vi "LS370Monitor.vi"() -> ()   [LabVIEW 2019]
uses:
  Utility/LS370/Monitor/LS370_Status.ctl
  Instrument_Setup.vi
  Global/Global Variables/global.vi
  Global/Global Variables/Data_Display_global.vi
  Utility/Monitor Communication/sub-vis/LS370_Open_Queue.vi
panel:
  out "Lakeshore 370":T1
  out "Tsweeps Running":bool
  in  "Stopp":bool
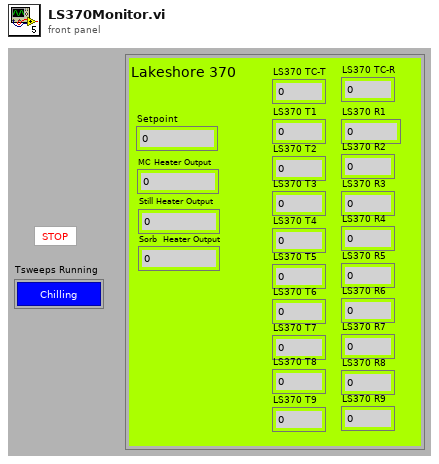
[diagram p1: front panel]
types:
  T1 = typedef "LS370_Status.ctl" = cluster{"Setpoint":dbl, "MC Heater Output":dbl, "Still Heater Output":dbl, "Sorb  Heater Output":dbl, "LS370 T1":dbl, "LS370 T2":dbl, "LS370 T3":dbl, "LS370 T4":dbl, "LS370 T5":dbl, "LS370 R1":dbl, "LS370 R2":dbl, "LS370 R3":dbl, "LS370 R4":dbl, "LS370 R5":dbl, "LS370 T6":dbl, "LS370 T7":dbl, "LS370 T8":dbl, "LS370 T9":dbl, "LS370 R6":dbl, "LS370 R7":dbl, "LS370 R8":dbl, "LS370 R9":dbl, "LS370 TC-T":dbl, "LS370 TC-R":dbl}
  T2 = typedef "LS370-Control.ctl" = cluster{"Disable Heater":bool, "Activate Tsweep":bool, "Update Lakeshores":bool, "Setpoint - Manual":dbl, "Rate (K/min)":dbl, "Sorb Power (mW)":dbl, "Still Power (mW)":dbl, "Sorb Heater":bool, "Still Heater":bool, "Set Temperature Sweep Main":bool}
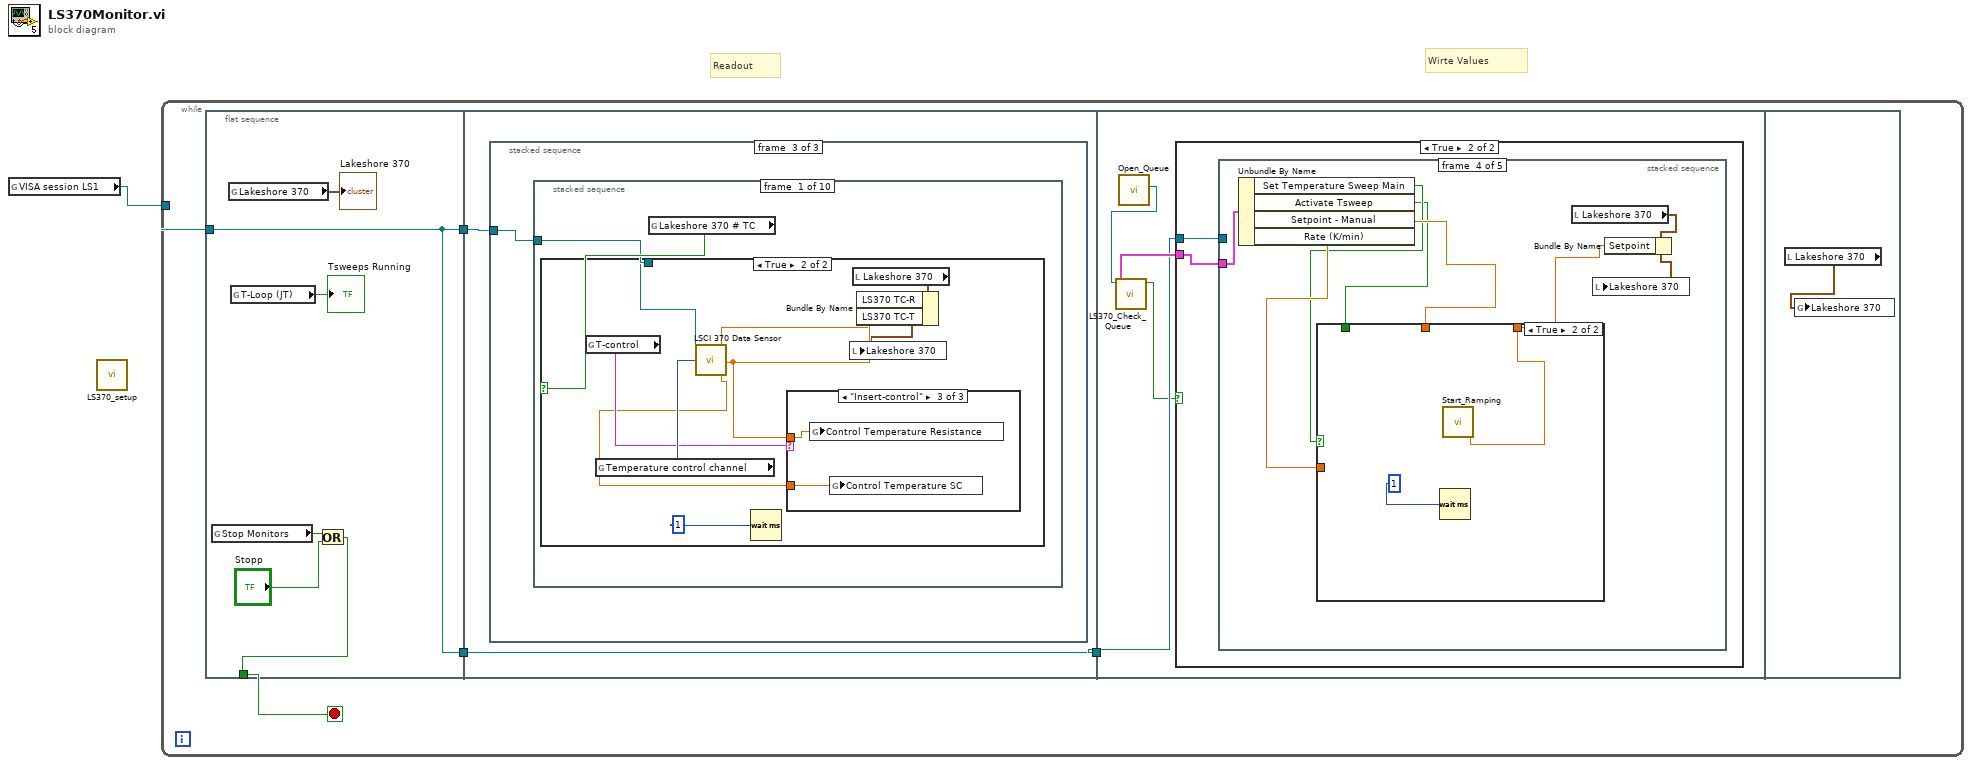
[diagram p0: block diagram]
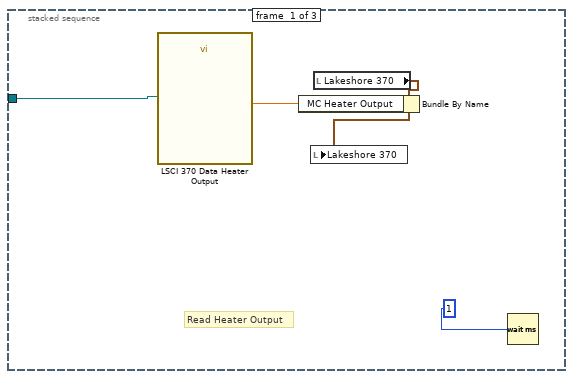
[diagram p2: hidden frame]
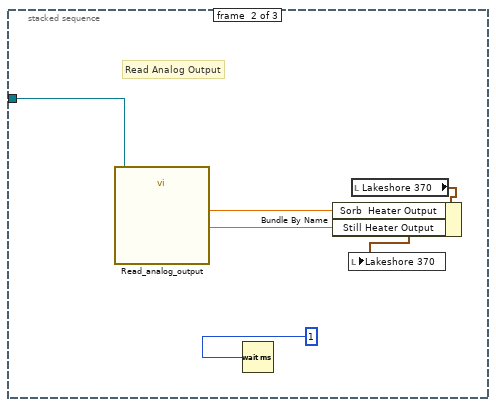
[diagram p3: hidden frame]
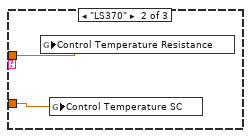
[diagram p6: hidden frame]
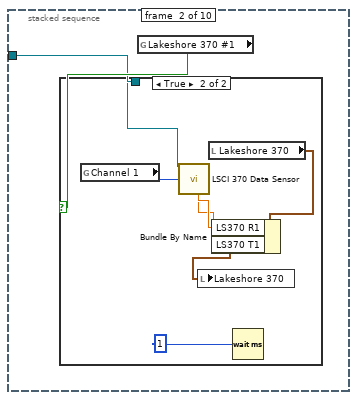
[diagram p7: hidden frame]
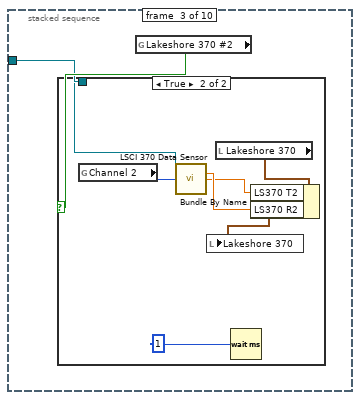
[diagram p9: hidden frame]
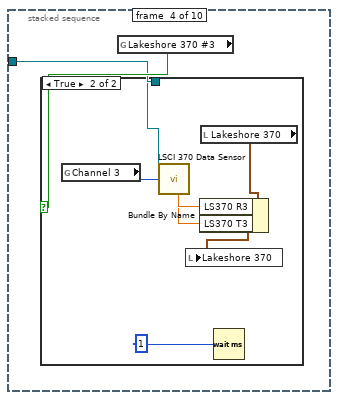
[diagram p11: hidden frame]
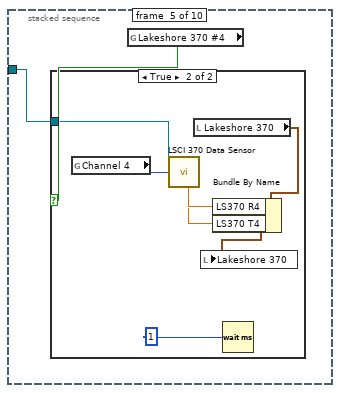
[diagram p13: hidden frame]
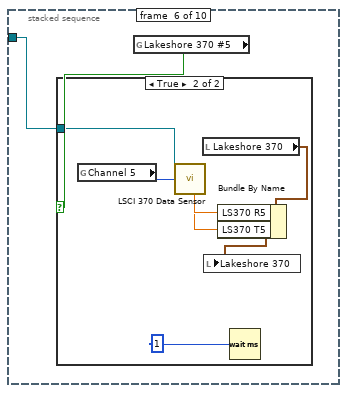
[diagram p15: hidden frame]
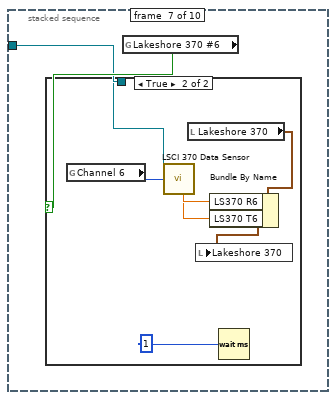
[diagram p17: hidden frame]
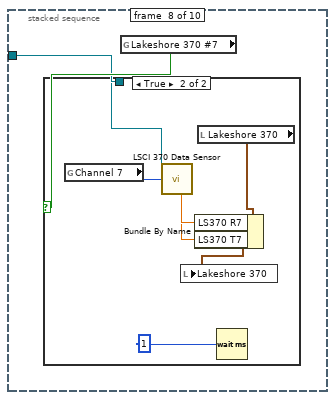
[diagram p19: hidden frame]
diagram:
  # "Wirte Values"
  # "Readout"
  n1 = global read "Instrument_Setup.vi" "VISA session LS1"() -> (w1:refnum<visa-resource-name>)
  n2 = call "LS370_setup.vi"() -> ()  [unwired: 1 in]
  n3 = while {
    tunnel: w1 -> [w5]
    stop <- w2 stop-if-true
    n4 = flat-sequence {
      tunnel: w5 -> [w8]
      tunnel: [w8] -> w6
      tunnel: [w8] -> w3
      tunnel: [w7] -> w2
      tunnel: w6 -> [w14]
      tunnel: [w13] -> w4
      tunnel: w3 -> [w13]
      tunnel: w4 -> [w124]
      frame #0 {
        n5 = global read "Data_Display_global.vi" "Stop Monitors"() -> (w10:bool)
        n6 = global read "Data_Display_global.vi" "Lakeshore 370"() -> (→"Lakeshore 370":T1)
        n7 = global read "global.vi" "T-Loop (JT)"() -> (→"Tsweeps Running":bool)
        n8 = Or(x=w10, y="Stopp") -> (x .or. y?=w7:bool)
      }
      frame #1 {
        n9 = stacked-sequence {
          tunnel: w14 -> [w19 w25 w26]
          frame #0 {
            # "Read Heater Output"
            n10 = call "LSCI 370 Data Heater Output.vi"("VISA session"=w19) -> ("Heater Output"=w16:dbl)  [unwired: 12 in, 2 out]
            n11 = local read "Lakeshore 370"() -> (w17:T1)
            n12 = Bundle By Name(cluster=w17, "MC Heater Output"=w16) -> (w15:T1)
            n13 = local write "Lakeshore 370"(w15) -> ()
            n14 = Wait (ms)(milliseconds to wait=1) -> ()  [unwired: 1 out]
          }
          frame #1 {
            # "Read Analog Output"
            n15 = call "Read_analog_output.vi"("VISA session"=w25) -> ("Still Output"=w20:dbl, "Analog Output"=w21:dbl)  [unwired: 9 in]
            n16 = Wait (ms)(milliseconds to wait=1) -> ()  [unwired: 1 out]
            n17 = local read "Lakeshore 370"() -> (w23:T1)
            n18 = Bundle By Name(cluster=w23, "Sorb  Heater Output"=w21, "Still Heater Output"=w20) -> (w22:T1)
            n19 = local write "Lakeshore 370"(w22) -> ()
          }
          frame #2 {
            n20 = stacked-sequence {
              tunnel: w26 -> [w27 w41 w50 w59 w68 w77 w86 w95 w104 w113]
              frame #0 {
                n21 = global read "Instrument_Setup.vi" "Lakeshore 370 # TC"() -> (w28:bool)
                n22 = case shown="True" w28 {
                  tunnel: w27 -> [_ w34]
                  frame False {
                  }
                  frame True {
                    n23 = global read "Instrument_Setup.vi" "T-control"() -> (w33:string)
                    n24 = global read "Instrument_Setup.vi" "Temperature control channel"() -> (w36:i32)
                    n25 = call "LSCI 370 Data Sensor.vi"("VISA session"=w34, "Channel (1)"=w36) -> ("Resistance Reading"=w31:dbl, "Kelvin Reading"=w30:dbl)  [unwired: 9 in, 3 out]
                    n26 = Wait (ms)(milliseconds to wait=1) -> ()  [unwired: 1 out]
                    n27 = case shown="\"Insert-control\"" w33 {
                      tunnel: w31 -> [_ w38 w40]
                      tunnel: w30 -> [_ w37 w39]
                      frame "None", Default {
                      }
                      frame "LS370" {
                        n28 = global write "Data_Display_global.vi" "Control Temperature Resistance"(w38) -> ()
                        n29 = global write "Data_Display_global.vi" "Control Temperature SC"(w37) -> ()
                      }
                      frame "Insert-control" {
                        n30 = global write "Data_Display_global.vi" "Control Temperature Resistance"(w40) -> ()
                        n31 = global write "Data_Display_global.vi" "Control Temperature SC"(w39) -> ()
                      }
                    }
                    n32 = local read "Lakeshore 370"() -> (w32:T1)
                    n33 = Bundle By Name(cluster=w32, "LS370 TC-R"=w31, "LS370 TC-T"=w30) -> (w29:T1)
                    n34 = local write "Lakeshore 370"(w29) -> ()
                  }
                }
              }
              frame #1 {
                n35 = global read "Instrument_Setup.vi" "Lakeshore 370 #1"() -> (w42:bool)
                n36 = case shown="True" w42 {
                  tunnel: w41 -> [_ w47]
                  frame False {
                  }
                  frame True {
                    n37 = global read "Instrument_Setup.vi" "Channel 1"() -> (w49:i32)
                    n38 = call "LSCI 370 Data Sensor.vi"("VISA session"=w47, "Channel (1)"=w49) -> ("Resistance Reading"=w44:dbl, "Kelvin Reading"=w43:dbl)  [unwired: 9 in, 3 out]
                    n39 = local read "Lakeshore 370"() -> (w46:T1)
                    n40 = Bundle By Name(cluster=w46, "LS370 R1"=w44, "LS370 T1"=w43) -> (w45:T1)
                    n41 = local write "Lakeshore 370"(w45) -> ()
                    n42 = Wait (ms)(milliseconds to wait=1) -> ()  [unwired: 1 out]
                  }
                }
              }
              frame #2 {
                n43 = global read "Instrument_Setup.vi" "Lakeshore 370 #2"() -> (w51:bool)
                n44 = case shown="True" w51 {
                  tunnel: w50 -> [_ w56]
                  frame False {
                  }
                  frame True {
                    n45 = global read "Instrument_Setup.vi" "Channel 2"() -> (w58:i32)
                    n46 = call "LSCI 370 Data Sensor.vi"("VISA session"=w56, "Channel (1)"=w58) -> ("Resistance Reading"=w53:dbl, "Kelvin Reading"=w52:dbl)  [unwired: 9 in, 3 out]
                    n47 = local read "Lakeshore 370"() -> (w55:T1)
                    n48 = Wait (ms)(milliseconds to wait=1) -> ()  [unwired: 1 out]
                    n49 = Bundle By Name(cluster=w55, "LS370 T2"=w52, "LS370 R2"=w53) -> (w54:T1)
                    n50 = local write "Lakeshore 370"(w54) -> ()
                  }
                }
              }
              frame #3 {
                n51 = global read "Instrument_Setup.vi" "Lakeshore 370 #3"() -> (w60:bool)
                n52 = case shown="True" w60 {
                  tunnel: w59 -> [_ w65]
                  frame False {
                  }
                  frame True {
                    n53 = global read "Instrument_Setup.vi" "Channel 3"() -> (w67:i32)
                    n54 = call "LSCI 370 Data Sensor.vi"("VISA session"=w65, "Channel (1)"=w67) -> ("Resistance Reading"=w62:dbl, "Kelvin Reading"=w61:dbl)  [unwired: 9 in, 3 out]
                    n55 = local read "Lakeshore 370"() -> (w64:T1)
                    n56 = Bundle By Name(cluster=w64, "LS370 R3"=w62, "LS370 T3"=w61) -> (w63:T1)
                    n57 = local write "Lakeshore 370"(w63) -> ()
                    n58 = Wait (ms)(milliseconds to wait=1) -> ()  [unwired: 1 out]
                  }
                }
              }
              frame #4 {
                n59 = global read "Instrument_Setup.vi" "Lakeshore 370 #4"() -> (w69:bool)
                n60 = case shown="True" w69 {
                  tunnel: w68 -> [_ w74]
                  frame False {
                  }
                  frame True {
                    n61 = global read "Instrument_Setup.vi" "Channel 4"() -> (w76:i32)
                    n62 = call "LSCI 370 Data Sensor.vi"("VISA session"=w74, "Channel (1)"=w76) -> ("Resistance Reading"=w71:dbl, "Kelvin Reading"=w70:dbl)  [unwired: 9 in, 3 out]
                    n63 = local read "Lakeshore 370"() -> (w73:T1)
                    n64 = Bundle By Name(cluster=w73, "LS370 R4"=w71, "LS370 T4"=w70) -> (w72:T1)
                    n65 = local write "Lakeshore 370"(w72) -> ()
                    n66 = Wait (ms)(milliseconds to wait=1) -> ()  [unwired: 1 out]
                  }
                }
              }
              frame #5 {
                n67 = global read "Instrument_Setup.vi" "Lakeshore 370 #5"() -> (w78:bool)
                n68 = case shown="True" w78 {
                  tunnel: w77 -> [_ w83]
                  frame False {
                  }
                  frame True {
                    n69 = global read "Instrument_Setup.vi" "Channel 5"() -> (w85:i32)
                    n70 = call "LSCI 370 Data Sensor.vi"("VISA session"=w83, "Channel (1)"=w85) -> ("Resistance Reading"=w81:dbl, "Kelvin Reading"=w80:dbl)  [unwired: 9 in, 3 out]
                    n71 = local read "Lakeshore 370"() -> (w82:T1)
                    n72 = Bundle By Name(cluster=w82, "LS370 R5"=w81, "LS370 T5"=w80) -> (w79:T1)
                    n73 = local write "Lakeshore 370"(w79) -> ()
                    n74 = Wait (ms)(milliseconds to wait=1) -> ()  [unwired: 1 out]
                  }
                }
              }
              frame #6 {
                n75 = global read "Instrument_Setup.vi" "Lakeshore 370 #6"() -> (w87:bool)
                n76 = case shown="True" w87 {
                  tunnel: w86 -> [_ w92]
                  frame False {
                  }
                  frame True {
                    n77 = global read "Instrument_Setup.vi" "Channel 6"() -> (w94:i32)
                    n78 = call "LSCI 370 Data Sensor.vi"("VISA session"=w92, "Channel (1)"=w94) -> ("Resistance Reading"=w90:dbl, "Kelvin Reading"=w89:dbl)  [unwired: 9 in, 3 out]
                    n79 = local read "Lakeshore 370"() -> (w91:T1)
                    n80 = Bundle By Name(cluster=w91, "LS370 R6"=w90, "LS370 T6"=w89) -> (w88:T1)
                    n81 = local write "Lakeshore 370"(w88) -> ()
                    n82 = Wait (ms)(milliseconds to wait=1) -> ()  [unwired: 1 out]
                  }
                }
              }
              frame #7 {
                n83 = global read "Instrument_Setup.vi" "Lakeshore 370 #7"() -> (w96:bool)
                n84 = case shown="True" w96 {
                  tunnel: w95 -> [_ w101]
                  frame False {
                  }
                  frame True {
                    n85 = global read "Instrument_Setup.vi" "Channel 7"() -> (w103:i32)
                    n86 = call "LSCI 370 Data Sensor.vi"("VISA session"=w101, "Channel (1)"=w103) -> ("Resistance Reading"=w99:dbl, "Kelvin Reading"=w98:dbl)  [unwired: 9 in, 3 out]
                    n87 = local read "Lakeshore 370"() -> (w100:T1)
                    n88 = Bundle By Name(cluster=w100, "LS370 R7"=w99, "LS370 T7"=w98) -> (w97:T1)
                    n89 = local write "Lakeshore 370"(w97) -> ()
                    n90 = Wait (ms)(milliseconds to wait=1) -> ()  [unwired: 1 out]
                  }
                }
              }
              frame #8 {
                n91 = global read "Instrument_Setup.vi" "Lakeshore 370 #8"() -> (w105:bool)
                n92 = case shown="True" w105 {
                  tunnel: w104 -> [_ w110]
                  frame False {
                  }
                  frame True {
                    n93 = global read "Instrument_Setup.vi" "Channel 8"() -> (w112:i32)
                    n94 = call "LSCI 370 Data Sensor.vi"("VISA session"=w110, "Channel (1)"=w112) -> ("Resistance Reading"=w108:dbl, "Kelvin Reading"=w107:dbl)  [unwired: 9 in, 3 out]
                    n95 = local read "Lakeshore 370"() -> (w109:T1)
                    n96 = Bundle By Name(cluster=w109, "LS370 R8"=w108, "LS370 T8"=w107) -> (w106:T1)
                    n97 = local write "Lakeshore 370"(w106) -> ()
                    n98 = Wait (ms)(milliseconds to wait=1) -> ()  [unwired: 1 out]
                  }
                }
              }
              frame #9 {
                n99 = global read "Instrument_Setup.vi" "Lakeshore 370 #9"() -> (w114:bool)
                n100 = case shown="True" w114 {
                  tunnel: w113 -> [_ w119]
                  frame False {
                  }
                  frame True {
                    n101 = global read "Instrument_Setup.vi" "Channel 9"() -> (w121:i32)
                    n102 = call "LSCI 370 Data Sensor.vi"("VISA session"=w119, "Channel (1)"=w121) -> ("Resistance Reading"=w117:dbl, "Kelvin Reading"=w116:dbl)  [unwired: 9 in, 3 out]
                    n103 = local read "Lakeshore 370"() -> (w118:T1)
                    n104 = Bundle By Name(cluster=w118, "LS370 R9"=w117, "LS370 T9"=w116) -> (w115:T1)
                    n105 = local write "Lakeshore 370"(w115) -> ()
                    n106 = Wait (ms)(milliseconds to wait=1) -> ()  [unwired: 1 out]
                  }
                }
              }
            }
          }
        }
      }
      frame #2 {
        n107 = call-poly "Open_Queue.vi"() -> ("queue out"=w123:refnum<queue>)  [unwired: 10 in, 1 out]
        n108 = call "LS370_Check_Queue.vi"("queue"=w123) -> ("Control"=w125:T2, "New Entries?"=w122:bool)  [unwired: 7 in, 1 out]
        n109 = case shown="True" w122 {
          tunnel: w125 -> [_ w126]
          tunnel: w124 -> [_ w127]
          frame False {
          }
          frame True {
            n110 = stacked-sequence {
              tunnel: w127 -> [w133 w139 _ _ _]
              tunnel: w126 -> [w130 w136 w141 w150 w166]
              frame #0 {
                # "Set Still Power"
                n111 = global read "Instrument_Setup.vi" "Still Heater Resistance (Analog  Out  2)"() -> (w132:dbl)
                n112 = Unbundle By Name(w130) -> ("Still Heater"=w129:bool, "Still Power (mW)"=w128:dbl)
                n113 = call "Set_Still_Power.vi"("VISA session"=w133, "Still Heater Resistance (mW)"=w132, "Still Power (mW)"=w128, "Still heater"=w129) -> ()  [unwired: 8 in]
                n114 = Wait (ms)(milliseconds to wait=1) -> ()  [unwired: 1 out]
              }
              frame #1 {
                # "Set Sorb Power"
                n115 = Unbundle By Name(w136) -> ("Sorb Heater"=w134:bool, "Sorb Power (mW)"=w135:dbl)
                n116 = global read "Instrument_Setup.vi" "Sorb Heater Resistance (Analog Out 1)"() -> (w138:dbl)
                n117 = call "Set_Sorb_Power.vi"("VISA session"=w139, "Sorb Heater Resistance (Ohm)"=w138, "Sorb Power (mW)"=w135, "Sorb heater"=w134) -> ()  [unwired: 8 in]
                n118 = Wait (ms)(milliseconds to wait=1) -> ()  [unwired: 1 out]
              }
              frame #2 {
                n119 = Unbundle By Name(w141) -> ("Update Lakeshores"=w140:bool)
                n120 = case shown="True" w140 {
                  frame False {
                  }
                  frame True {
                    n121 = flat-sequence {
                      frame #0 {
                        n122 = call "LS370_setup.vi"() -> ()  [unwired: 1 in]
                        n123 = Wait (ms)(milliseconds to wait=1) -> ()  [unwired: 1 out]
                      }
                    }
                  }
                }
              }
              frame #3 {
                n124 = Unbundle By Name(w150) -> ("Set Temperature Sweep Main"=w144:bool, "Activate Tsweep"=w143:bool, "Setpoint - Manual"=w148:dbl, "Rate (K/min)"=w149:dbl)
                n125 = case shown="True" w144 {
                  tunnel: [w154 w163] -> w145
                  tunnel: w149 -> [w153 _]
                  tunnel: w143 -> [w152 _]
                  tunnel: w148 -> [w151 _]
                  frame False {
                    n126 = case shown="False" w152 {
                      tunnel: w151 -> [_ w161]
                      tunnel: w153 -> [_ w162]
                      tunnel: [w155 w161] -> w154
                      frame False {
                        n127 = global read "global.vi" "Cerrent State"() -> (w158:i32)
                        n128 = Equal?(x=1, y=w158) -> (x = y?=w156:bool)
                        n129 = case shown="False" w156 {
                          tunnel: [w159 w160] -> w155
                          frame False {
                            n130 = global read "global.vi" "T final (K)"() -> (w159:dbl)
                          }
                          frame True {
                            n131 = global read "global.vi" "T init. (K)"() -> (w160:dbl)
                          }
                        }
                      }
                      frame True {
                        n132 = call "Start_Sweep_Manual.vi"("Rate"=w162, "Setpoint"=w161) -> ()  [unwired: 10 in]
                      }
                    }
                  }
                  frame True {
                    n133 = Wait (ms)(milliseconds to wait=1) -> ()  [unwired: 1 out]
                    n134 = call "Start_Ramping.vi"() -> ("Setpoint"=w163:dbl)  [unwired: 11 in]
                  }
                }
                n135 = local read "Lakeshore 370"() -> (w147:T1)
                n136 = Bundle By Name(cluster=w147, "Setpoint"=w145) -> (w146:T1)
                n137 = local write "Lakeshore 370"(w146) -> ()
              }
              frame #4 {
                n138 = Unbundle By Name(w166) -> ("Disable Heater"=w165:bool)
                n139 = case shown="True" w165 {
                  frame False {
                  }
                  frame True {
                    n140 = call "Disable_Zone_Tuning.vi"() -> ()  [unwired: 1 in]
                    n141 = Wait (ms)(milliseconds to wait=10) -> ()  [unwired: 1 out]
                  }
                }
              }
            }
          }
        }
      }
      frame #3 {
        n142 = local read "Lakeshore 370"() -> (w168:T1)
        n143 = global write "Data_Display_global.vi" "Lakeshore 370"(w168) -> ()
      }
    }
  }
